vi "CLC_GEN4_L2_InPhaseCal_mW_BackUP.vi"() -> ()   [LabVIEW 2023, in "Clover_Cell.lvlib"]
uses:
  Clover_Cell.lvlib
  lib/Anritsu Signal Analyzer Series/Anritsu Signal Analyzer Series.lvlib
  lib/ELTA/ELTA.lvlib
panel:
  out "Total mW":dbl format="%.7f"
  out "Total dBm":dbl format="%.7f"
  out "Ref. mW":dbl format="%.7f"
  out "Ref. dBm":dbl format="%.7f"
  out "Main mW":dbl format="%.7f"
  out "Main dBm":dbl format="%.7f"
  out "Data":dbl[][](array[numeric])
  out "FileNAME_Single":string
  in  "VISA resource name":refnum<visa-resource-name>="TCPIP0::192.168.100.230::inst0::INSTR"
  in  "CenterFreq(GHz)":dbl=27.0
  out "PhaseStep":i32=63
  in  "AvgTimes":i32=3
  out "SA1":dbl[](graph)
  out "CurrentData":dbl[](array[numeric])
  out "Duration":dbl
  in  "Single_Channel_Phase_Sweep":bool
  out "TotalTime":dbl format="%.2f"
  out "StopTime":timestamp=timestamp(3663835912.033212 s since 1904-01-01)
  out "FileNAME_Dual":string
  out "StartTime":timestamp=timestamp(3663835741.875155 s since 1904-01-01)
  out "trmode":u16=1
  in  "TRXmode":u16(ring)=1 items=["Rx"=2, "Tx"=1]
  out "error out":errorcluster
  out "output cluster":T1={"address"="192.168.100.111", "remote port or service name"=5025, "timeout ms (60000)"=10000}
  out "Operating \nChannel(s)":bool[][](array[boolean])
  in  "Polarity":u16(ring) items=["V", "H"]
  out "Channel":i32=63
  out "OK?":bool
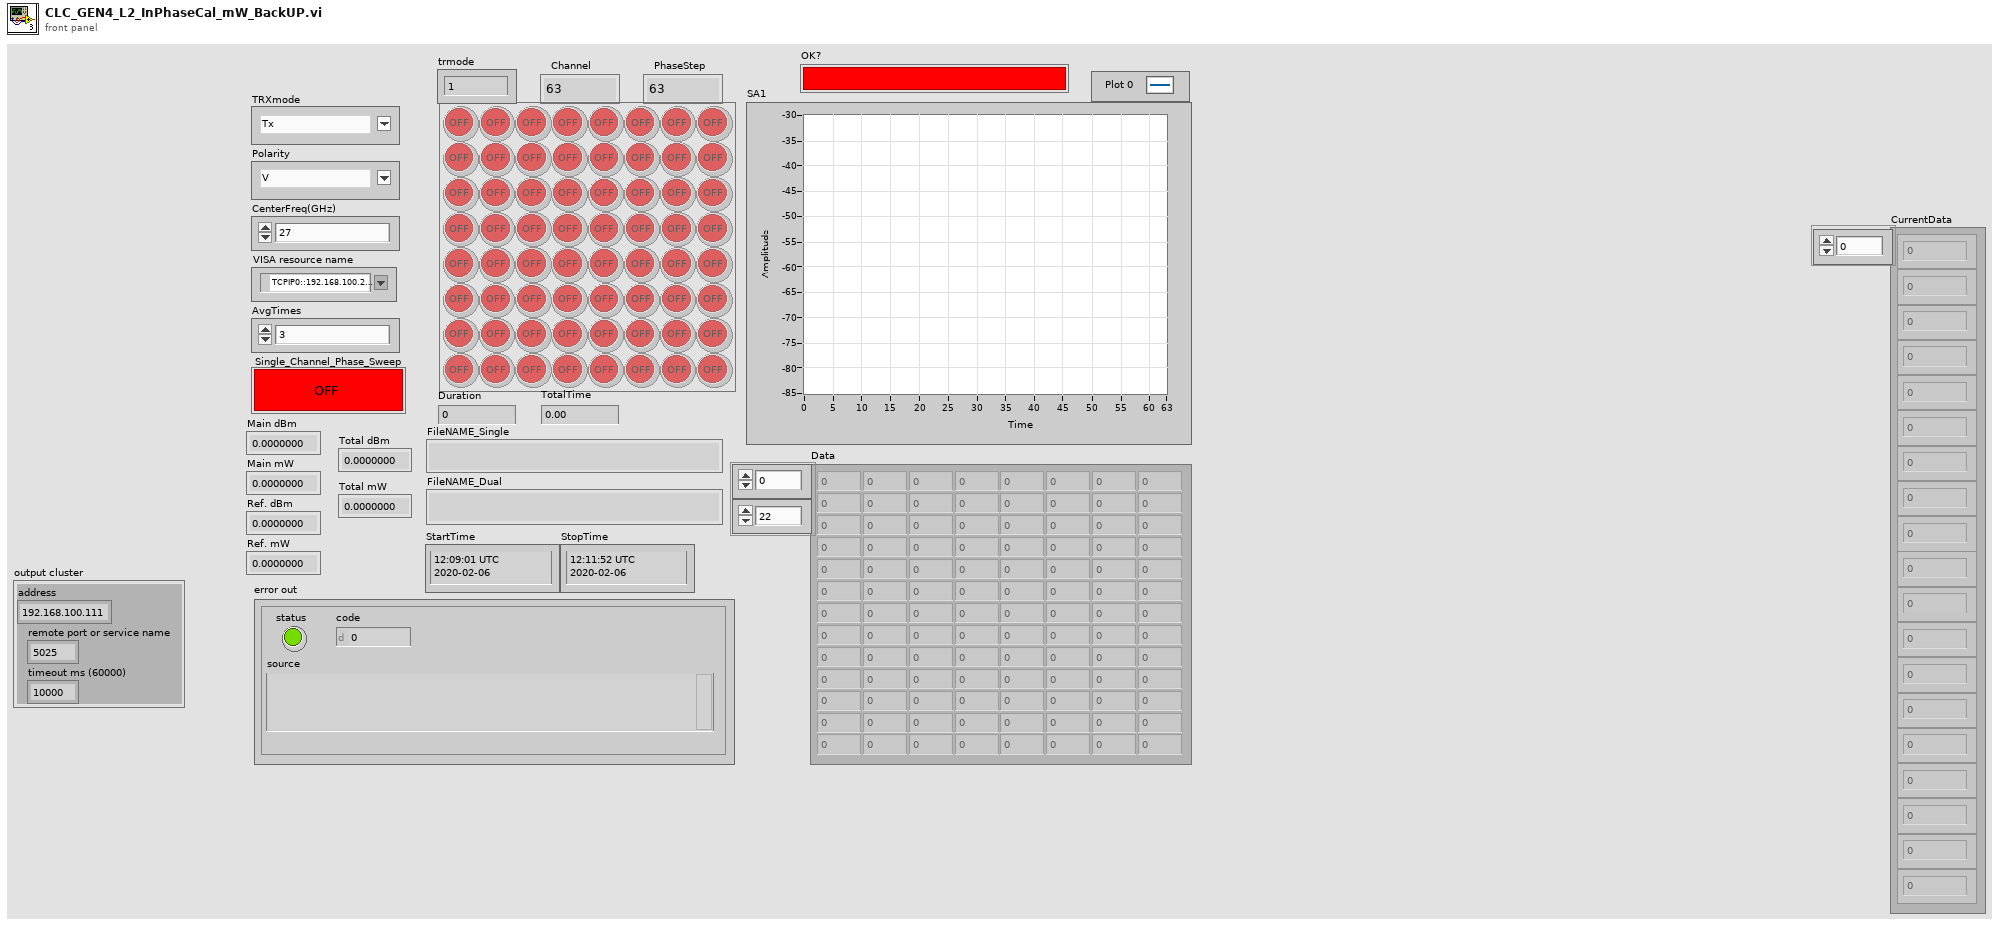
[diagram p1: front panel]
types:
  T1 = cluster{"address":string, "remote port or service name":u16, "timeout ms (60000)":i32}
  T2 = cluster{"Mode":u16, "Polarity":u16, "CH_ON/OFF":u16, "Channel":i32, "Gain":i32, "Phase":i32}
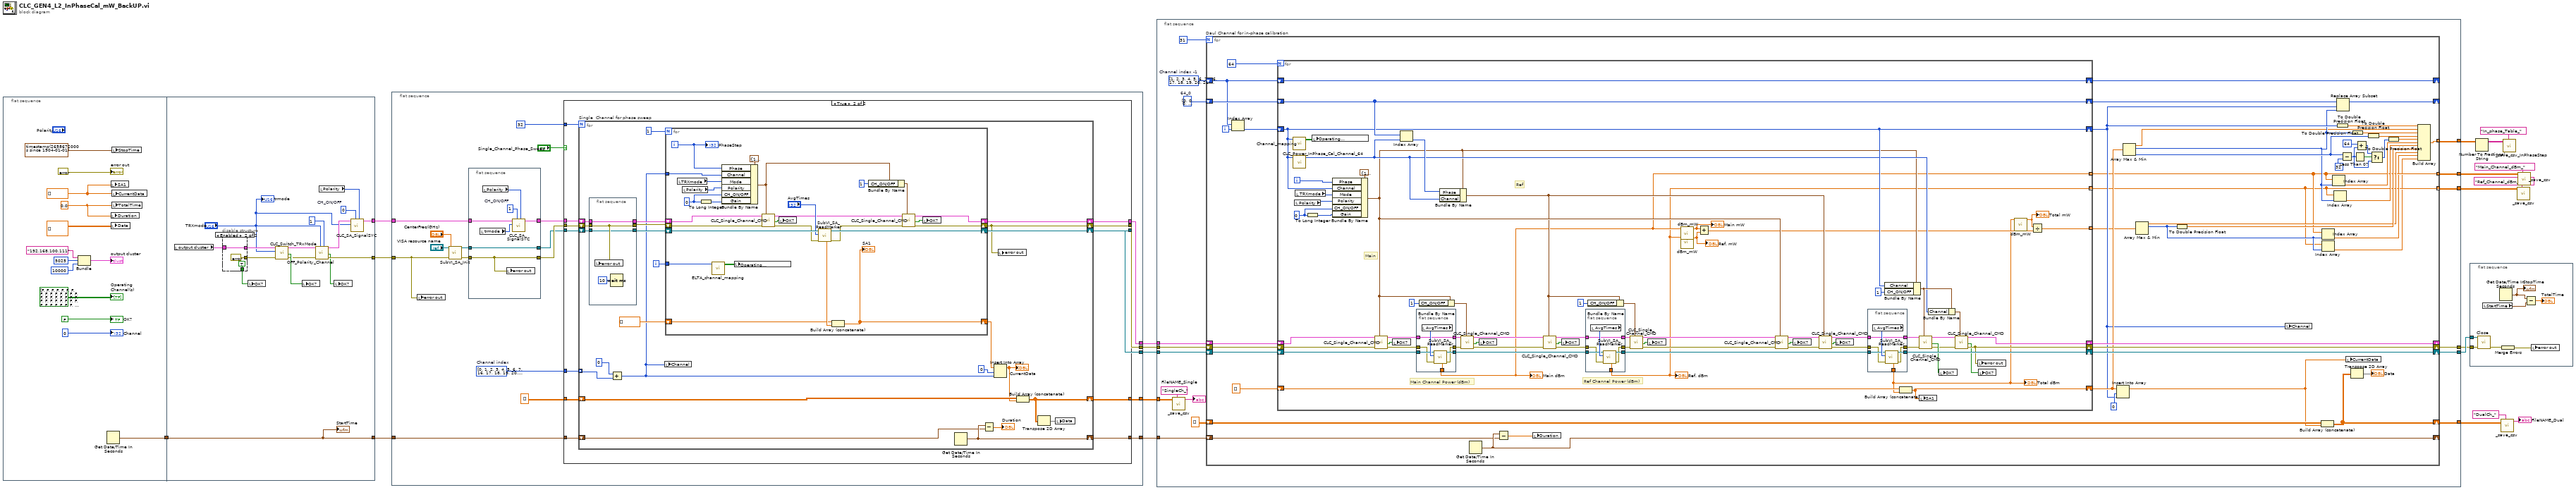
[diagram p0: block diagram]
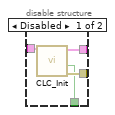
[diagram p3: hidden frame]
diagram:
  n1 = flat-sequence {
    tunnel: [w22] -> w21
    tunnel: w21 -> [w38]
    tunnel: [w41] -> w8
    tunnel: [w45] -> w10
    tunnel: [w38] -> w20
    frame #0 {
      w26 = dbl[] []
      w29 = 0.0 ("TotalTime")
      n2 = Bundle("address"="192.168.100.111", "remote port or service name"=u16 5025, "timeout ms (60000)"=10000) -> (→"output cluster":T1)  [unwired: 1 in]
      n3 = Get Date/Time In Seconds() -> (seconds since 1Jan1904=w22:timestamp)
      n4 = local write "SA1"(w26) -> ()
      n5 = local write "Duration"(w29) -> ()
      n6 = local write "Data"(dbl[][] []) -> ()
      n7 = local write "StopTime"(timestamp(2658672000.001 s since 1904-01-01) ("StopTime")) -> ()
      n8 = local write "CurrentData"(w26) -> ()
      n9 = local write "TotalTime"(w29) -> ()
      "error out" <- errorcluster {"status"=FALSE, "code"=0, "source"=""} ("error out")
      "Operating \nChannel(s)" <- bool[][] [[FALSE, FALSE, FALSE, FALSE, FALSE, FALSE, FALSE, FALSE], [FALSE, FALSE, FALSE, FALSE, FALSE, FALSE, FALSE, FALSE], [FALSE, FALSE, FALSE, FALSE, FALSE, FALSE, FALSE, FALSE], [FALSE, FALSE, FALSE, FALSE, FALSE, FALSE, FALSE, FALSE], [FALSE, FALSE, FALSE, FALSE, FALSE, FALSE, FALSE, FALSE], [FALSE, FALSE, FALSE, FALSE, FALSE, FALSE, FALSE, FALSE], [FALSE, FALSE, FALSE, FALSE, FALSE, FALSE, FALSE, FALSE], [FALSE, FALSE, FALSE, FALSE, FALSE, FALSE, FALSE, FALSE]] ("Operating \nChannel(s)")
      "Channel" <- 0 ("Channel")
      "OK?" <- FALSE ("OK?")
    }
    frame #1 {
      w40 = u16 0  # CH_ON/OFF
      n10 = local read "output cluster"() -> (w50:T1)
      n11 = disable-structure shown="Enabled" {
        disable-tunnel: w50 -> [w54 w57]
        disable-tunnel: [w53 w57] -> w49
        disable-tunnel: [w52 errorcluster {"status"=FALSE, "code"=0, "source"=""} ("error in (no error)")] -> w47
        disable-tunnel: [w51 TRUE ("OK?")] -> w39
        frame Disabled {
          n12 = call "CLC_Init.vi"("TCPIPin"=w54) -> ("error out"=w52:errorcluster, "Status"=w51:bool, "TCPIPin 2"=w53:T1)  [unwired: 8 in]
        }
        frame Enabled {
        }
      }
      n13 = local write "OK?"(w39) -> ()
      n14 = call "CLC_Switch_TRxMode.vi"("error in (no error)"=w47, "Text Ring"="TRXmode", "TCPIPin"=w49) -> ("error out"=w46:errorcluster, "OK?"=w48:bool, "TCPIPin 2"=w44:T1)  [unwired: 6 in]
      n15 = local write "OK?"(w48) -> ()
      n16 = call "OFF_Polarity_Channel.vi"("CH_ON:0/OFF:1"=u16 1, "Mode"="TRXmode", "error in"=w46, "TCPIPin"=w44) -> ("error out"=w45:errorcluster, "OK?"=w43:bool, "TCPIPout"=w42:T1)  [unwired: 5 in]
      n17 = local read "Polarity"() -> (w36:u16)
      n18 = local write "OK?"(w43) -> ()
      n19 = call "CLC_SA_SignalSYC.vi"("Polarity"=w36, "CH_ON/OFF"=w40, "Mode"="TRXmode", "TCPIPin"=w42) -> ("TCPIPout"=w41:T1)  [unwired: 7 in]
      "StartTime" <- w38
      "trmode" <- "TRXmode"
    }
  }
  n20 = flat-sequence {
    tunnel: w20 -> [w74]
    tunnel: [w73] -> w19
    tunnel: [w72] -> w18
    tunnel: [w71] -> w17
    tunnel: [w70] -> w11
    tunnel: w10 -> [w68]
    tunnel: w8 -> [w63]
    tunnel: [w58] -> w7
    frame #0 {
      w65 = i32[] [0, 1, 2, 3, 4, 5, 6, 7, 16, 17, 18, 19, 20, 21, 22, 23, 32, 33, 34, 35, 36, 37, 38, 39, 48, 49, 50, 51, 52, 53, 54, 55]  # Channel index
      n21 = local write "error out"(w68) -> ()
      n22 = call "SubVI_SA_Init.vi"("error in (no error)"=w68, "CenterFreq(GHz) 2"="CenterFreq(GHz)", "VISA resource name"="VISA resource name") -> ("error out 2"=w69:errorcluster, "VISA resource name out"=w62:refnum<visa-resource-name>)  [unwired: 6 in, 1 out]
      n23 = flat-sequence {
        tunnel: w69 -> [w155]
        tunnel: [w155] -> w64
        tunnel: w63 -> [w153]
        tunnel: w62 -> [w154]
        tunnel: [w154] -> w61
        tunnel: [w152] -> w60
        frame #0 {
          w151 = u16 1  # CH_ON/OFF
          n24 = local read "trmode"() -> (w149:u16)
          n25 = local read "Polarity"() -> (w150:u16)
          n26 = local write "error out"(w155) -> ()
          n27 = call "CLC_SA_SignalSYC.vi"("Polarity"=w150, "CH_ON/OFF"=w151, "Mode"=w149, "TCPIPin"=w153) -> ("TCPIPout"=w152:T1)  [unwired: 7 in]
        }
      }
      n28 = case shown="True" "Single_Channel_Phase_Sweep" {
        tunnel: [w78 w93] -> w58
        tunnel: 32 -> [_ w92]
        tunnel: w74 -> [w77 w91]
        tunnel: [w79 w90] -> w73
        tunnel: [w80 w89] -> w72
        tunnel: [w81 w88] -> w71
        tunnel: [w77 w87] -> w70
        tunnel: dbl[][] [] -> [w78 w86]
        tunnel: w65 -> [_ w85]
        tunnel: w64 -> [w80 w84]
        tunnel: w61 -> [w79 w83]
        tunnel: w60 -> [w81 w82]
        frame False {
        }
        frame True {
          n29 = for "Single  Channel for phase sweep" {
            N: w92 -> [_]
            shift-right: [w117] -> w88
            shift-left: w82 -> [w101]
            shift-right: [w111] -> w89
            shift-left: w84 -> [w103]
            shift-right: [w115] -> w90
            shift-left: w83 -> [w100]
            shift-right: [w109] -> w93
            shift-left: w86 -> [w110]
            shift-right: [w113] -> w87
            shift-left: w91 -> [w112]
            tunnel: w85 -> [w97] mode=indexing
            i -> [w96]
            n30 = flat-sequence {
              tunnel: [w119] -> w99
              tunnel: w103 -> [w120]
              tunnel: [w120] -> w102
              tunnel: w101 -> [w119]
              tunnel: w100 -> [w118]
              tunnel: [w118] -> w98
              frame #0 {
                n31 = local write "error out"(w120) -> ()
                n32 = Wait (ms)(milliseconds to wait=u32 10) -> ()  [unwired: 1 out]
              }
            }
            n33 = Add(x=0, y=w97) -> (x+y=w95:i32)
            n34 = local write "Channel"(w95) -> ()
            n35 = for {
              N: 1 -> [_]
              shift-right: [w128] -> w117
              shift-left: w99 -> [w140]
              shift-right: [w130] -> w111
              shift-left: w102 -> [w142]
              shift-right: [w147] -> w115
              shift-left: w98 -> [w148]
              shift-right: [w143] -> w108
              shift-left: dbl[] [] -> [w144]
              tunnel: w95 -> [w137]
              tunnel: w96 -> [w123]
              i -> [w133]
              w134 = u16 0 ("CH_ON/OFF")
              n36 = local read "TRXmode"() -> (w136:u16)
              n37 = local read "Polarity"() -> (w135:u16)
              n38 = To Long Integer(number=w134) -> (32bit integer=w132:i32)
              n39 = call "ELTA_channel_mapping.vi"("Channel IN"=w123) -> ("Operating \nChannel(s)"=w122:bool[][])  [unwired: 10 in]
              n40 = Bundle By Name(cluster=T2 {"Mode"=1, "Polarity"=1, "CH_ON/OFF"=1, "Channel"=0, "Gain"=0, "Phase"=0} ("Channel params"), "Phase"=w133, "Channel"=w137, "Mode"=w136, "Polarity"=w135, "CH_ON/OFF"=w134, "Gain"=w132) -> (w127:T2)
              n41 = local write "Operating \nChannel(s)"(w122) -> ()
              n42 = call "CLC_Single_Channel_CMD.vi"("Channel params"=w127, "error in"=w142, "TCPIPin"=w140) -> ("error out"=w141:errorcluster, "OK?"=w138:bool, "TCPIPout"=w129:T1)  [unwired: 6 in]
              n43 = local write "OK?"(w138) -> ()
              n44 = call "SubVI_SA_ReadMarker.vi"("error in (no error)"=w141, "AvgTimes"="AvgTimes", "VISA resource name"=w148) -> ("error out"=w131:errorcluster, "VISA resource name out"=w147:refnum<visa-resource-name>, "Marker Power"=w145:dbl)  [unwired: 5 in, 1 out]
              n45 = Build Array (concatenate)(w144, w145) -> (w143:dbl[])
              "SA1" <- w143
              n46 = Bundle By Name(cluster=w127, "CH_ON/OFF"=u16 1) -> (w125:T2)
              n47 = call "CLC_Single_Channel_CMD.vi"("Channel params"=w125, "error in"=w131, "TCPIPin"=w129) -> ("error out"=w130:errorcluster, "OK?"=w124:bool, "TCPIPout"=w128:T1)  [unwired: 6 in]
              n48 = local write "OK?"(w124) -> ()
              "PhaseStep" <- w133
            }
            n49 = Get Date/Time In Seconds() -> (seconds since 1Jan1904=w113:timestamp)
            n50 = Subtract(x=w113, y=w112) -> (x-y=→"Duration":dbl)
            n51 = Insert Into Array(array=w108, index=0, new element=w95) -> (w105:dbl[])
            "CurrentData" <- w105
            n52 = local write "error out"(w111) -> ()
            n53 = Build Array (concatenate)(w110, w105) -> (w109:dbl[][])
            n54 = Transpose 2D Array(2D array=w109) -> (transposed array=w94:dbl[][])
            n55 = local write "Data"(w94) -> ()
          }
        }
      }
    }
  }
  n56 = flat-sequence {
    tunnel: w19 -> [w171]
    tunnel: w18 -> [w170]
    tunnel: w17 -> [w169]
    tunnel: [w168] -> w14
    tunnel: [w167] -> w13
    tunnel: [w166] -> w12
    tunnel: w11 -> [w165]
    tunnel: [w163] -> w6
    tunnel: w7 -> [w161]
    tunnel: [w157] -> w4
    tunnel: [w156] -> w2
    frame #0 {
      w158 = i32[] [0, 0, 0, 0, 0, 0, 0, 0, 0, 0, 0, 0, 0, 0, 0, 0, 0, 0, 0, 0, 0, 0, 0, 0, 0, 0, 0, 0, 0, 0, 0, 0, 0, 0, 0, 0, 0, 0, 0, 0, 0, 0, 0, 0, 0, 0, 0, 0, 0, 0, 0, 0, 0, 0, 0, 0, 0, 0, 0, 0, 0, 0, 0, 0]  # 64_0
      w162 = i32[] [1, 2, 3, 4, 5, 6, 7, 16, 17, 18, 19, 20, 21, 22, 23, 32, 33, 34, 35, 36, 37, 38, 39, 48, 49, 50, 51, 52, 53, 54, 55]  # Channel index -1
      n57 = call "_save_csv.vi"("delimiter (\\t)"="SingleCh_" ("delimiter (\\t)"), "Data"=w161) -> ("FileName"=→"FileNAME_Single":string)  [unwired: 9 in]
      n58 = for "Daul Channel for in-phase calibration" {
        N: 31 -> [_]
        shift-right: [w221] -> _
        shift-left: w169 -> [w206]
        shift-right: [w218] -> w166
        shift-left: w170 -> [w207]
        shift-right: [w219] -> w167
        shift-left: w171 -> [w217]
        shift-right: [w212] -> w168
        shift-left: dbl[][] [] -> [w213]
        shift-right: [w216] -> _
        shift-left: w165 -> [w215]
        shift-right: [w191] -> _
        shift-left: w158 -> [w202]
        tunnel: [w204] -> w163 mode=indexing
        shift-right: [w201] -> _
        shift-left: w162 -> [w200]
        tunnel: [w177] -> w157 mode=indexing
        tunnel: [w174] -> w156 mode=indexing
        i -> [w203]
        n59 = Index Array(array=w200, index=w203) -> (element=w199:i32)
        n60 = for {
          N: 64 -> [_]
          shift-right: [w264] -> w221
          shift-left: w206 -> [w254]
          shift-right: [w268] -> w218
          shift-left: w207 -> [w255]
          shift-right: [w288] -> w219
          shift-left: w217 -> [w253]
          shift-right: [w260] -> w205
          shift-left: dbl[] [] -> [w287]
          shift-right: [w275] -> w190
          shift-left: w202 -> [w275]
          shift-right: [w262] -> w201
          shift-left: w200 -> [w262]
          shift-right: [w259] -> w189
          shift-left: w199 -> [w259]
          tunnel: [w228] -> w177 mode=indexing
          tunnel: [w225] -> w174 mode=indexing
          tunnel: [w227] -> w188 mode=indexing
          i -> [w281]
          w285 = u16 0 ("CH_ON/OFF")
          # "Ref Channel Power (dBm)"
          # "Main Channel Power (dBm)"
          # "Ref"
          # "Main"
          n61 = call "Channel_mapping.vi"("Channel IN"=w259) -> ("Operating \nChannel(s)"=w263:bool[][])  [unwired: 10 in]
          n62 = call "CLC_Power_InPhase_Cal_Channel_64.vi"("Channel IN"=w259) -> ("Ref_Channel"=w258:i32)  [unwired: 8 in, 2 out]
          n63 = local read "Polarity"() -> (w284:u16)
          n64 = local read "TRXmode"() -> (w283:u16)
          n65 = To Long Integer(number=w285) -> (32bit integer=w286:i32)
          n66 = local write "Operating \nChannel(s)"(w263) -> ()
          n67 = Bundle By Name(cluster=T2 {"Mode"=1, "Polarity"=1, "CH_ON/OFF"=1, "Channel"=0, "Gain"=0, "Phase"=0} ("Channel params"), "Phase"=w281, "Channel"=w259, "Mode"=w283, "Polarity"=w284, "CH_ON/OFF"=w285, "Gain"=w286) -> (w250:T2)
          n68 = call "CLC_Single_Channel_CMD.vi"("Channel params"=w250, "error in"=w255, "TCPIPin"=w254) -> ("error out"=w252:errorcluster, "OK?"=w257:bool, "TCPIPout"=w251:T1)  [unwired: 6 in]
          n69 = local write "OK?"(w257) -> ()
          n70 = Index Array(array=w275, index=w258) -> (element=w274:i32)
          n71 = flat-sequence {
            tunnel: [w302] -> w234
            tunnel: [w300] -> w228
            tunnel: w253 -> [w299]
            tunnel: w252 -> [w298]
            tunnel: [w297] -> w245
            tunnel: w251 -> [w297]
            tunnel: [w296] -> w246
            frame #0 {
              n72 = local read "AvgTimes"() -> (w301:i32)
              n73 = call "SubVI_SA_ReadMarker.vi"("error in (no error)"=w298, "AvgTimes"=w301, "VISA resource name"=w299) -> ("error out"=w296:errorcluster, "VISA resource name out"=w302:refnum<visa-resource-name>, "Marker Power"=w300:dbl)  [unwired: 5 in, 1 out]
            }
          }
          n74 = Bundle By Name(cluster=w250, "CH_ON/OFF"=u16 1) -> (w247:T2)
          n75 = Bundle By Name(cluster=w250, "Phase"=w274, "Channel"=w258) -> (w230:T2)
          n76 = call "CLC_Single_Channel_CMD.vi"("Channel params"=w247, "error in"=w246, "TCPIPin"=w245) -> ("error out"=w232:errorcluster, "OK?"=w249:bool, "TCPIPout"=w231:T1)  [unwired: 6 in]
          n77 = local write "OK?"(w249) -> ()
          n78 = call "CLC_Single_Channel_CMD.vi"("Channel params"=w230, "error in"=w232, "TCPIPin"=w231) -> ("error out"=w238:errorcluster, "OK?"=w237:bool, "TCPIPout"=w239:T1)  [unwired: 6 in]
          n79 = local write "OK?"(w237) -> ()
          n80 = flat-sequence {
            tunnel: [w295] -> w233
            tunnel: [w293] -> w225
            tunnel: w234 -> [w292]
            tunnel: w238 -> [w291]
            tunnel: [w290] -> w244
            tunnel: w239 -> [w290]
            tunnel: [w289] -> w243
            frame #0 {
              n81 = local read "AvgTimes"() -> (w294:i32)
              n82 = call "SubVI_SA_ReadMarker.vi"("error in (no error)"=w291, "AvgTimes"=w294, "VISA resource name"=w292) -> ("error out"=w289:errorcluster, "VISA resource name out"=w295:refnum<visa-resource-name>, "Marker Power"=w293:dbl)  [unwired: 5 in, 1 out]
            }
          }
          n83 = Bundle By Name(cluster=w230, "CH_ON/OFF"=u16 1) -> (w242:T2)
          n84 = call "CLC_Single_Channel_CMD.vi"("Channel params"=w242, "error in"=w243, "TCPIPin"=w244) -> ("error out"=w235:errorcluster, "OK?"=w240:bool, "TCPIPout"=w236:T1)  [unwired: 6 in]
          n85 = local write "OK?"(w240) -> ()
          n86 = call "dBm_mW.vi"("dBm"=w228) -> ("mW"=w226:dbl)  [unwired: 10 in]
          "Main mW" <- w226
          n87 = call "dBm_mW.vi"("dBm"=w225) -> ("mW"=w224:dbl)  [unwired: 10 in]
          "Ref. mW" <- w224
          n88 = Add(x=w226, y=w224) -> (x+y=w229:dbl)
          n89 = call "CLC_Single_Channel_CMD.vi"("Channel params"=w250, "error in"=w235, "TCPIPin"=w236) -> ("error out"=w279:errorcluster, "OK?"=w278:bool, "TCPIPout"=w280:T1)  [unwired: 6 in]
          n90 = local write "OK?"(w278) -> ()
          n91 = call "CLC_Single_Channel_CMD.vi"("Channel params"=w230, "error in"=w279, "TCPIPin"=w280) -> ("error out"=w276:errorcluster, "OK?"=w277:bool, "TCPIPout"=w273:T1)  [unwired: 6 in]
          n92 = local write "OK?"(w277) -> ()
          n93 = flat-sequence {
            tunnel: [w309] -> w288
            tunnel: [w307] -> w223
            tunnel: w233 -> [w306]
            tunnel: w276 -> [w305]
            tunnel: [w304] -> w272
            tunnel: w273 -> [w304]
            tunnel: [w303] -> w256
            frame #0 {
              n94 = local read "AvgTimes"() -> (w308:i32)
              n95 = call "SubVI_SA_ReadMarker.vi"("error in (no error)"=w305, "AvgTimes"=w308, "VISA resource name"=w306) -> ("error out"=w303:errorcluster, "VISA resource name out"=w309:refnum<visa-resource-name>, "Marker Power"=w307:dbl)  [unwired: 5 in, 1 out]
            }
          }
          n96 = Bundle By Name(cluster=w250, "Channel"=w259, "CH_ON/OFF"=u16 1) -> (w261:T2)
          n97 = Build Array (concatenate)(w287, w223) -> (w260:dbl[])
          n98 = call "CLC_Single_Channel_CMD.vi"("Channel params"=w261, "error in"=w256, "TCPIPin"=w272) -> ("error out"=w269:errorcluster, "OK?"=w270:bool, "TCPIPout"=w267:T1)  [unwired: 6 in]
          n99 = local write "SA1"(w260) -> ()
          n100 = Bundle By Name(cluster=w261, "Channel"=w258) -> (w266:T2)
          n101 = local write "OK?"(w270) -> ()
          n102 = call "CLC_Single_Channel_CMD.vi"("Channel params"=w266, "error in"=w269, "TCPIPin"=w267) -> ("error out"=w268:errorcluster, "OK?"=w265:bool, "TCPIPout"=w264:T1)  [unwired: 6 in]
          n103 = local write "error out"(w268) -> ()
          n104 = local write "OK?"(w265) -> ()
          n105 = call "dBm_mW.vi"("dBm"=w223) -> ("mW"=w222:dbl)  [unwired: 10 in]
          "Total mW" <- w222
          n106 = Divide(x=w222, y=w229) -> (x/y=w227:dbl)
          "Main dBm" <- w228
          "Ref. dBm" <- w225
          "Total dBm" <- w223
        }
        n107 = Get Date/Time In Seconds() -> (seconds since 1Jan1904=w216:timestamp)
        n108 = Subtract(x=w216, y=w215) -> (x-y=w214:dbl)
        n109 = local write "Duration"(w214) -> ()
        n110 = Insert Into Array(array=w205, index=0, new element=w189) -> (w208:dbl[])
        n111 = Array Max & Min(array=w205) -> (max value=w181:dbl, max index (indices)=w184:i32, min index (indices)=w198:i32)  [unwired: 1 out]
        n112 = Array Max & Min(array=w188) -> (max value=w178:dbl, max index (indices)=w176:i32)  [unwired: 2 out]
        n113 = To Double Precision Float(number=w176) -> (double precision float=w179:dbl)
        n114 = local write "Channel"(w189) -> ()
        n115 = Build Array (concatenate)(w213, w208) -> (w212:dbl[][])
        n116 = Index Array(array=w177, index=w176) -> (element=w175:dbl)
        n117 = Index Array(array=w174, index=w176) -> (element=w173:dbl)
        n118 = Index Array(array=w177, index=w184) -> (element=w183:dbl)
        n119 = Index Array(array=w174, index=w184) -> (element=w182:dbl)
        n120 = To Double Precision Float(number=w189) -> (double precision float=w180:dbl)
        n121 = Replace Array Subset(array=w190, new element=w184, index=w189) -> (w191:i32[])
        n122 = Subtract(x=w198, y=32) -> (x-y=w193:i32)
        n123 = local write "CurrentData"(w208) -> ()
        n124 = Transpose 2D Array(2D array=w212) -> (transposed array=→"Data":dbl[][])
        n125 = To Double Precision Float(number=w184) -> (double precision float=w187:dbl)
        n126 = Less Than 0?(x=w193) -> (x < 0?=w196:bool)
        n127 = Add(x=64, y=w193) -> (x+y=w194:i32)
        n128 = To Double Precision Float(number=w198) -> (double precision float=w186:dbl)
        n129 = Select(t=w194, s=w196, f=w193) -> (s? t:f=w192:i32)
        n130 = To Double Precision Float(number=w192) -> (double precision float=w185:dbl)
        n131 = Build Array(w180, w181, w187, w186, w185, w183, w182, w179, w178, w175, w173) -> (w204:dbl[])
      }
    }
  }
  n132 = flat-sequence {
    tunnel: w13 -> [w315]
    tunnel: w12 -> [w314]
    frame #0 {
      n133 = call "Close.vi"("error in (no error)"=w314, "VISA resource name"=w315) -> ("error out"=w316:errorcluster)  [unwired: 9 in]
      n134 = local read "StartTime"() -> (w310:timestamp)
      n135 = Get Date/Time In Seconds() -> (seconds since 1Jan1904=w311:timestamp)
      "StopTime" <- w311
      n136 = Merge Errors(w316) -> (w313:errorcluster)
      n137 = Subtract(x=w311, y=w310) -> (x-y=→"TotalTime":dbl)
      n138 = local write "error out"(w313) -> ()
    }
  }
  n139 = Number To Fractional String(number=w6) -> (F-format string=w1:string[][])  [unwired: 3 in]
  n140 = call "_save_csv.vi"("delimiter (\\t)"="DualCh_" ("delimiter (\\t)"), "Data"=w14) -> ("FileName"=→"FileNAME_Dual":string)  [unwired: 9 in]
  n141 = call "_save_csv_InPhaseStep.vi"("delimiter (\\t)"="In_phase_Table_" ("delimiter (\\t)"), "dataInput"=w1) -> ()  [unwired: 9 in, 1 out]
  n142 = call "_save_csv.vi"("delimiter (\\t)"="Ref_Channel_dBm_" ("delimiter (\\t)"), "Data"=w2) -> ()  [unwired: 9 in, 1 out]
  n143 = call "_save_csv.vi"("delimiter (\\t)"="Main_Channel_dBm_" ("delimiter (\\t)"), "Data"=w4) -> ()  [unwired: 9 in, 1 out]
